vi "11-type_analog_bis.vi"() -> ()   [LabVIEW 2017]
panel:
  out "Analog1":bool
  out ".not. x?":bool
  out "settings out":T1
  in  "settings in":T2={"Auto1"=TRUE, "Auto2"=TRUE, "Rel1"=TRUE, "Rel2"=TRUE, "Filt1"=TRUE, "Filt2"=TRUE, "Rate"=enum."Med", "Range1"=enum."10mV", "Range2"=enum."100mV", "Filt3"=TRUE, "Filt4"=TRUE, "Rel temp"=TRUE, "Analog1"=FALSE, "Analog2"=FALSE, "Analog temp"=FALSE, "Digital1"=TRUE, "Digital2"=TRUE, "Digital temp "=TRUE, "Window1"=enum."0,01%", "Window2"=enum."0,01%", "Window temp"=enum."0,01%", "RDGS1"="010", "RDGS2"="010", "RDGS temp"="010", "Type_type1"=TRUE, "Type_type2"=TRUE, "Type_type temp"=TRUE, "LSync"=FALSE, "Unit"=enum."C", "Sens"=TRUE, "Type tcoupl"=enum."J", "Junc"=TRUE, "prevState"=0}
  in  "this":i32
  out "next state":i32
  in  "button":i32
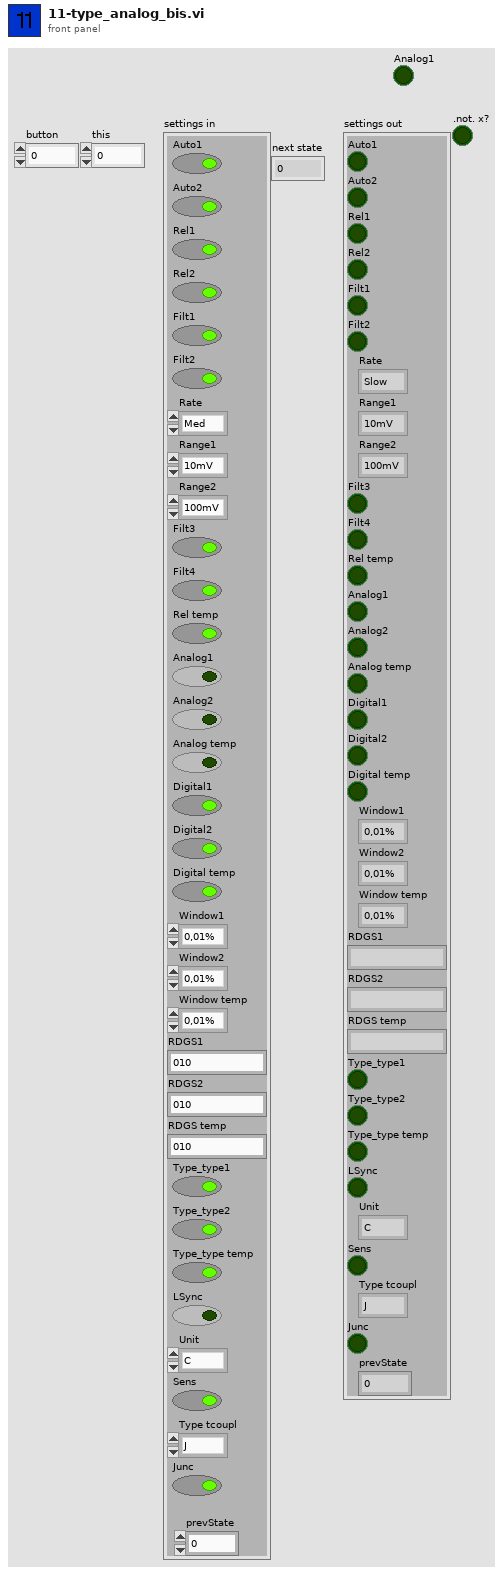
[diagram p1: front panel]
types:
  T1 = cluster{"Auto1":bool, "Auto2":bool, "Rel1":bool, "Rel2":bool, "Filt1":bool, "Filt2":bool, "Rate":enum16{"Slow", "Med", "Fast"}, "Range1":enum16{"10mV", "100mV", "1V", "10V", "100V"}, "Range2":enum16{"100mV", "1V", "10V"}, "Filt3":bool, "Filt4":bool, "Rel temp":bool, "Analog1":bool, "Analog2":bool, "Analog temp":bool, "Digital1":bool, "Digital2":bool, "Digital temp ":bool, "Window1":enum16{"0,01%", "0,1%", "1%", "10%", "None"}, "Window2":enum16{"0,01%", "0,1%", "1%", "10%", "None"}, "Window temp":enum16{"0,01%", "0,1%", "1%", "10%", "None"}, "RDGS1":string, "RDGS2":string, "RDGS temp":string, "Type_type1":bool, "Type_type2":bool, "Type_type temp":bool, "LSync":bool, "Unit":enum16{"C", "K", "F"}, "Sens":bool, "Type tcoupl":enum16{"J", "K", "T", "E", "R", "S", "B", "N"}, "Junc":bool, "prevState":dbl}
  T2 = cluster{"Auto1":bool, "Auto2":bool, "Rel1":bool, "Rel2":bool, "Filt1":bool, "Filt2":bool, "Rate":enum16{"Slow", "Med", "Fast"}, "Range1":enum16{"10mV", "100mV", "1V", "10V", "100V"}, "Range2":enum16{"100mV", "1V", "10V"}, "Filt3":bool, "Filt4":bool, "Rel temp":bool, "Analog1":bool, "Analog2":bool, "Analog temp":bool, "Digital1":bool, "Digital2":bool, "Digital temp ":bool, "Window1":enum16{"0,01%", "0,1%", "1%", "10%", "None"}, "Window2":enum16{"0,01%", "0,1%", "1%", "10%", "None"}, "Window temp":enum16{"0,01%", "0,1%", "1%", "10%", "None"}, "RDGS1":string, "RDGS2":string, "RDGS temp":string, "Type_type1":bool, "Type_type2":bool, "Type_type temp":bool, "LSync":bool, "Unit":enum16{"C", "K", "F"}, "Sens":bool, "Type tcoupl":enum16{"J", "K", "T", "E", "R", "S", "B", "N"}, "Junc":bool, "prevState":i32}
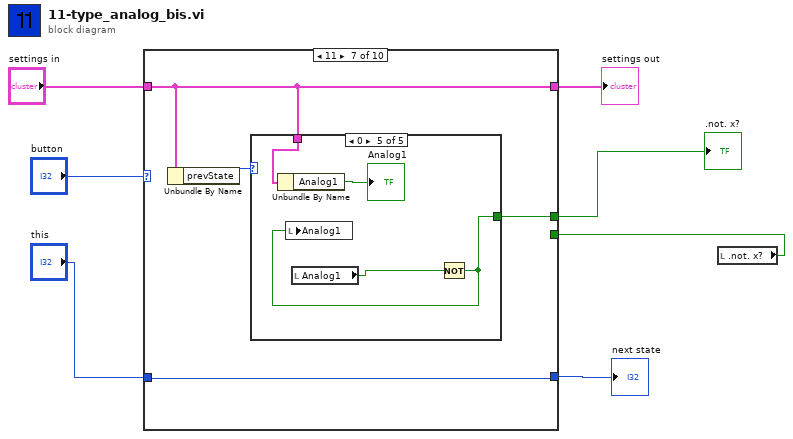
[diagram p0: block diagram]
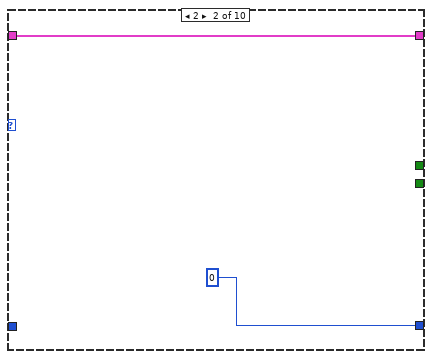
[diagram p3: hidden frame]
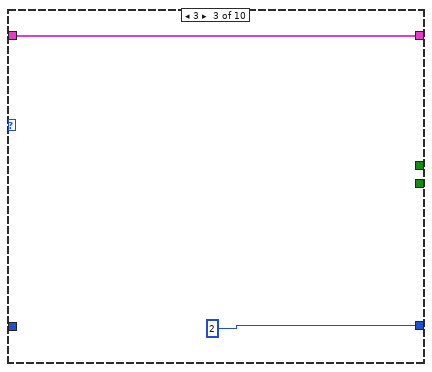
[diagram p4: hidden frame]
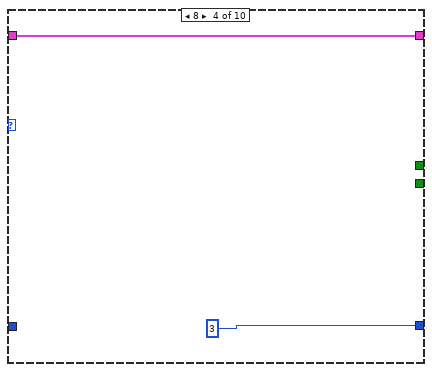
[diagram p5: hidden frame]
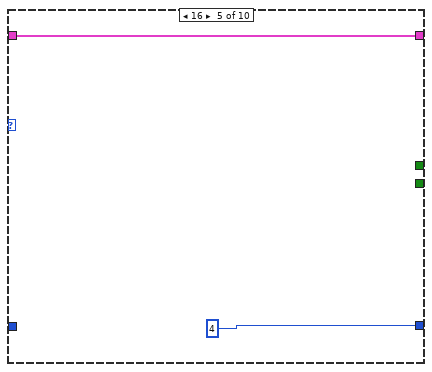
[diagram p6: hidden frame]
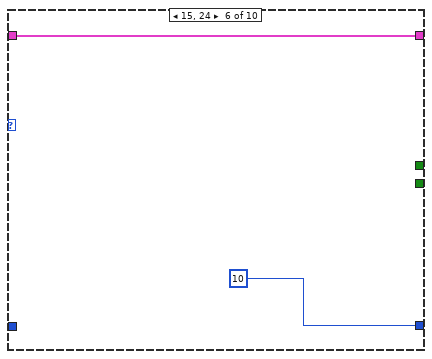
[diagram p7: hidden frame]
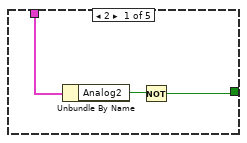
[diagram p8: hidden frame]
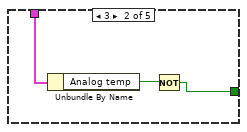
[diagram p9: hidden frame]
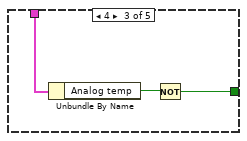
[diagram p10: hidden frame]
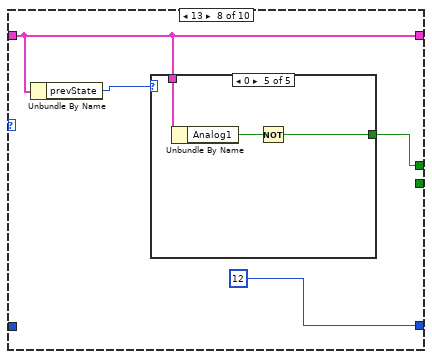
[diagram p12: hidden frame]
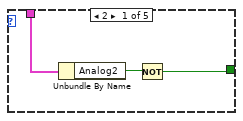
[diagram p13: hidden frame]
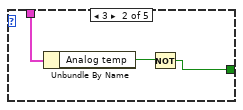
[diagram p14: hidden frame]
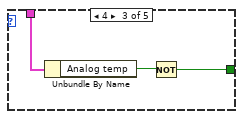
[diagram p15: hidden frame]
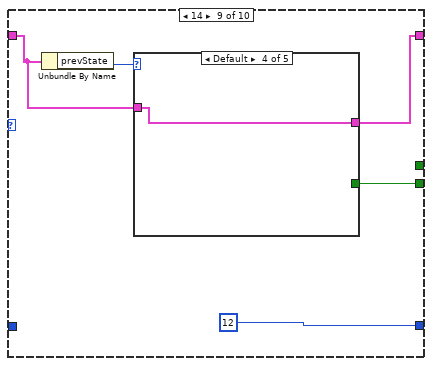
[diagram p17: hidden frame]
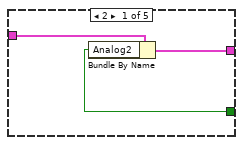
[diagram p18: hidden frame]
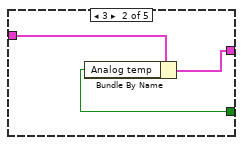
[diagram p19: hidden frame]
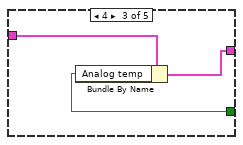
[diagram p20: hidden frame]
diagram:
  n1 = local read ".not. x?"() -> (w1:bool)
  n2 = case shown="11" "button" {
    tunnel: [w8 0 ("this") 2 3 4 10 ("this") w23 12 ("this") 12 ("this") w71] -> w3
    tunnel: "this" -> [w8 _ _ _ _ _ w23 _ _ _]
    tunnel: "settings in" -> [w9 w11 w12 w14 w16 w19 w21 w38 w54 w72]
    tunnel: [w9 w11 w12 w14 w16 w19 w21 w38 w55 w72] -> w4
    tunnel: [_ _ _ _ _ _ w20 w37 _ _] -> w2
    tunnel: w1 -> [_ _ _ _ _ _ _ _ w53 _]
    frame Default {
    }
    frame 2 {
    }
    frame 3 {
    }
    frame 8 {
    }
    frame 16 {
    }
    frame 15, 24 {
    }
    frame 11 {
      n3 = Unbundle By Name(w21) -> ("prevState"=w22:i32)
      n4 = case shown="0" w22 {
        tunnel: w21 -> [w26 w29 w31 _ w36]
        tunnel: [w24 w27 w30 _ w33] -> w20
        frame 2 {
          n5 = Unbundle By Name(w26) -> ("Analog2"=w25:bool)
          n6 = Not(x=w25) -> (.not. x?=w24:bool)
        }
        frame 3 {
          n7 = Unbundle By Name(w29) -> ("Analog temp"=w28:bool)
          n8 = Not(x=w28) -> (.not. x?=w27:bool)
        }
        frame 4 {
          n9 = Unbundle By Name(w31) -> ("Analog temp"=w32:bool)
          n10 = Not(x=w32) -> (.not. x?=w30:bool)
        }
        frame Default {
        }
        frame 0 {
          n11 = Unbundle By Name(w36) -> ("Analog1"=→"Analog1":bool)
          n12 = local read "Analog1"() -> (w34:bool)
          n13 = Not(x=w34) -> (.not. x?=w33:bool)
          n14 = local write "Analog1"(w33) -> ()
        }
      }
    }
    frame 13 {
      n15 = Unbundle By Name(w38) -> ("prevState"=w39:i32)
      n16 = case shown="0" w39 {
        tunnel: w38 -> [w43 w46 w48 _ w52]
        tunnel: [w41 w44 w47 _ w50] -> w37
        frame 2 {
          n17 = Unbundle By Name(w43) -> ("Analog2"=w42:bool)
          n18 = Not(x=w42) -> (.not. x?=w41:bool)
        }
        frame 3 {
          n19 = Unbundle By Name(w46) -> ("Analog temp"=w45:bool)
          n20 = Not(x=w45) -> (.not. x?=w44:bool)
        }
        frame 4 {
          n21 = Unbundle By Name(w48) -> ("Analog temp"=w49:bool)
          n22 = Not(x=w49) -> (.not. x?=w47:bool)
        }
        frame Default {
        }
        frame 0 {
          n23 = Unbundle By Name(w52) -> ("Analog1"=w51:bool)
          n24 = Not(x=w51) -> (.not. x?=w50:bool)
        }
      }
    }
    frame 14 {
      n25 = Unbundle By Name(w54) -> ("prevState"=w56:i32)
      n26 = case shown="Default" w56 {
        tunnel: [w59 w62 w65 w67 w70] -> w55
        tunnel: w54 -> [w60 w63 w66 w67 w69]
        tunnel: w53 -> [w58 w61 w64 _ w68]
        frame 2 {
          n27 = Bundle By Name(cluster=w60, "Analog2"=w58) -> (w59:T2)
        }
        frame 3 {
          n28 = Bundle By Name(cluster=w63, "Analog temp"=w61) -> (w62:T2)
        }
        frame 4 {
          n29 = Bundle By Name(cluster=w66, "Analog temp"=w64) -> (w65:T2)
        }
        frame Default {
        }
        frame 0 {
          n30 = Bundle By Name(cluster=w69, "Analog1"=w68) -> (w70:T2)
        }
      }
    }
    frame 32 {
      n31 = Unbundle By Name(w72) -> ("prevState"=w71:i32)
    }
  }
  "next state" <- w3
  "settings out" <- w4
  ".not. x?" <- w2
